vi "Initialise QuickDrop UI.vi"(5 "Type":T2=enum."Double Float", 7 "FP UI References":T1, 8 "error in (no error)":errorcluster) -> (0 "error out":errorcluster)   [LabVIEW 2016]
uses:
  <vilib>/Utility/Data Type/Type Definitions/Data Type.ctl
  FP UI References.ctl
  <vilib>/Utility/Data Type/NI_Data Type.lvlib
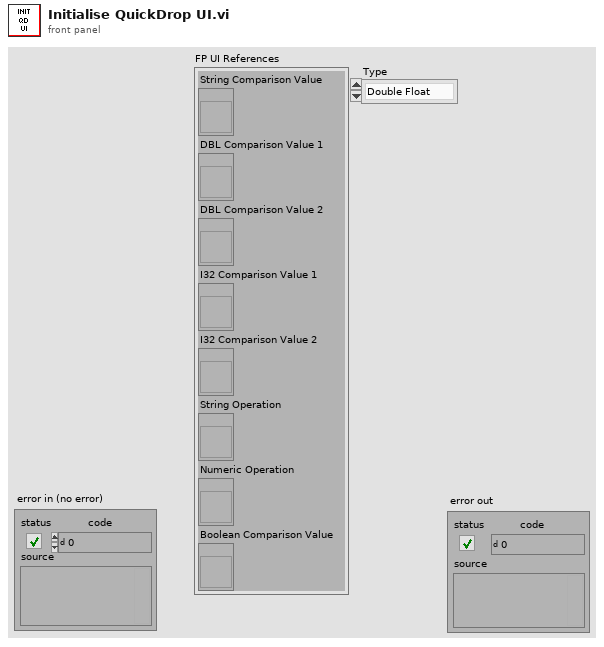
[diagram p1: front panel]
types:
  T1 = typedef "FP UI References.ctl" = cluster{"String Comparison Value":refnum<vi>, "DBL Comparison Value 1":refnum<vi>, "DBL Comparison Value 2":refnum<vi>, "I32 Comparison Value 1":refnum<vi>, "I32 Comparison Value 2":refnum<vi>, "String Operation":refnum<vi>, "Numeric Operation":refnum<vi>, "Boolean Comparison Value":refnum<vi>}
  T2 = typedef "NI_Data Type.lvlib/Data Type.ctl" = enum8{"Invalid Type", "Void", "I8", "I16", "I32", "I64", "U8", "U16", "U32", "U64", "Single Float", "Double Float", "Extended Float", "Single Complex", "Double Complex", "Extended Complex", "Enum U8", "Enum U16", "Enum U32", "Enum U64", "Single Float With Unit", "Double Float With Unit", "Extended Float With Unit", "Single Complex with Unit", "Double Complex with Unit", "Extended Complex with Unit", "Boolean", "String", "Path", "Picture", "Tag", "Array", "Cluster", "Variant", "LV Variant", "Waveform", "Timestamp", "Digital Waveform", "Digital Data", "ExpressData", "Refnum", "External Data", "VI", "Poly VI", "LabVIEW Class Instance", "Fixed Point"}
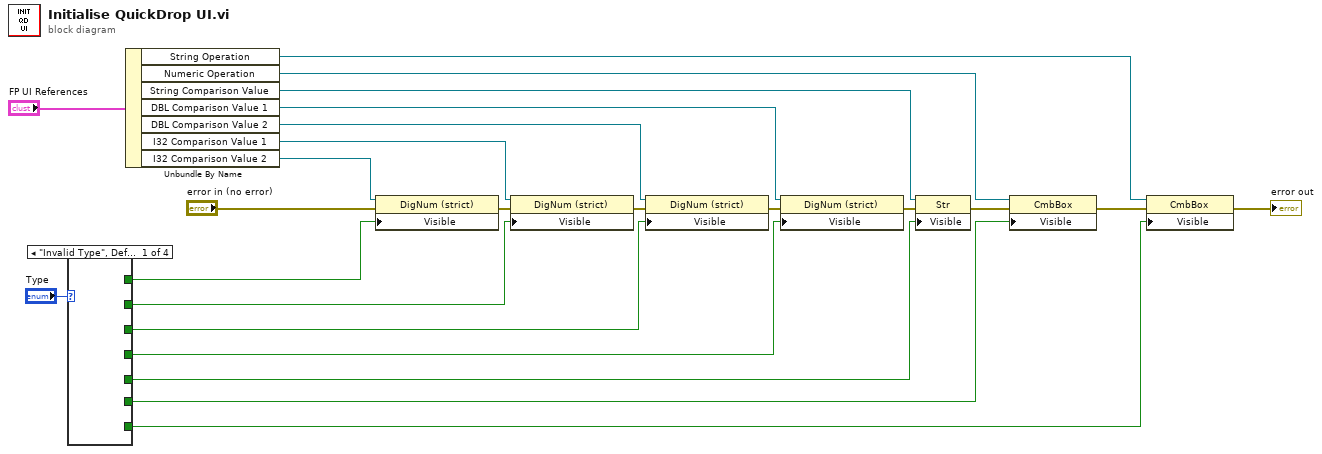
[diagram p0: block diagram]
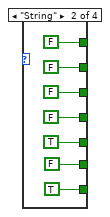
[diagram p2: hidden frame]
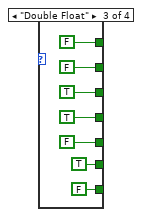
[diagram p3: hidden frame]
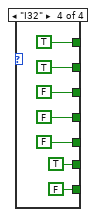
[diagram p4: hidden frame]
diagram:
  n1 = case shown="\"Invalid Type\", Default" "Type" {
    tunnel: [_ TRUE FALSE FALSE] -> w11
    tunnel: [_ FALSE TRUE FALSE] -> w7
    tunnel: [_ FALSE TRUE FALSE] -> w8
    tunnel: [_ FALSE FALSE TRUE] -> w9
    tunnel: [_ FALSE FALSE TRUE] -> w10
    tunnel: [_ TRUE FALSE FALSE] -> w2
    tunnel: [_ FALSE TRUE TRUE] -> w1
    frame "Invalid Type", Default {
    }
    frame "String" {
    }
    frame "Double Float" {
    }
    frame "I32" {
    }
  }
  n2 = Unbundle By Name("FP UI References") -> ("String Operation"=w3:refnum<vi>, "Numeric Operation"=w4:refnum<vi>, "String Comparison Value"=w22:refnum<vi>, "DBL Comparison Value 1"=w21:refnum<vi>, "DBL Comparison Value 2"=w20:refnum<vi>, "I32 Comparison Value 1"=w19:refnum<vi>, "I32 Comparison Value 2"=w18:refnum<vi>)
  n3 = property class="DigNum (strict)"(reference=w18, error in="error in (no error)", "Visible"=w10) -> (error out=w16:errorcluster)  [unwired: 1 out]
  n4 = property class="DigNum (strict)"(reference=w19, error in=w16, "Visible"=w9) -> (error out=w15:errorcluster)  [unwired: 1 out]
  n5 = property class="DigNum (strict)"(reference=w20, error in=w15, "Visible"=w8) -> (error out=w14:errorcluster)  [unwired: 1 out]
  n6 = property class="DigNum (strict)"(reference=w21, error in=w14, "Visible"=w7) -> (error out=w13:errorcluster)  [unwired: 1 out]
  n7 = property class="Str"(reference=w22, error in=w13, "Visible"=w11) -> (error out=w12:errorcluster)  [unwired: 1 out]
  n8 = property class="CmbBox"(reference=w4, error in=w12, "Visible"=w1) -> (error out=w6:errorcluster)  [unwired: 1 out]
  n9 = property class="CmbBox"(reference=w3, error in=w6, "Visible"=w2) -> (error out=→"error out":errorcluster)  [unwired: 1 out]
